vi "X682 Chassis Connectivity Tester Program Ver1.0.0.0.vi"() -> ()   [LabVIEW 2017]
uses:
  Ctrls/MainStep.ctl
  Ctrls/AllControls.ctl
  <vilib>/Utility/miscctls.llb/LVRowAndColumnTypeDef.ctl
  ComVIS/Files/Ini/WriteIniFiles_ByVarient.vi
  <instrlib>/GPP/GPP.lvlib
panel:
  in  "Recipe":string(combo)
  in  "MES Status":bool
  in  "maintenance":bool
  in  "mode":enum32{"Production mode", "Engineering mode"}(tab)
  out "Fail resume":bool caption="TotalResult"
  out "Table":string[][](table)
  out "LogInfo":string caption="Log"
  in  "AlarmData":i32(listbox)=-1
  out "Device state":bool caption="TotalResult"
  out "CT":dbl format="%#_3f"
  in  "ProductID:":string
  in  "TestInfo":T1 {"Yield" format="%#_g%"}
  out "MES_Status":string
  out "TestMode":string
  in  "Stop":bool
  in  "Start":bool
  in  "Exit":bool
  in  "Login":bool
  out "Login_status":string="Operator:Operator"
  out "OpenStatus":string
  in  "error in (no error)":errorcluster caption="错误输入（无错误）"
  # "Dyson X682 Chassis Connectivity Tester"
  # "Waiting Barcode scanning"
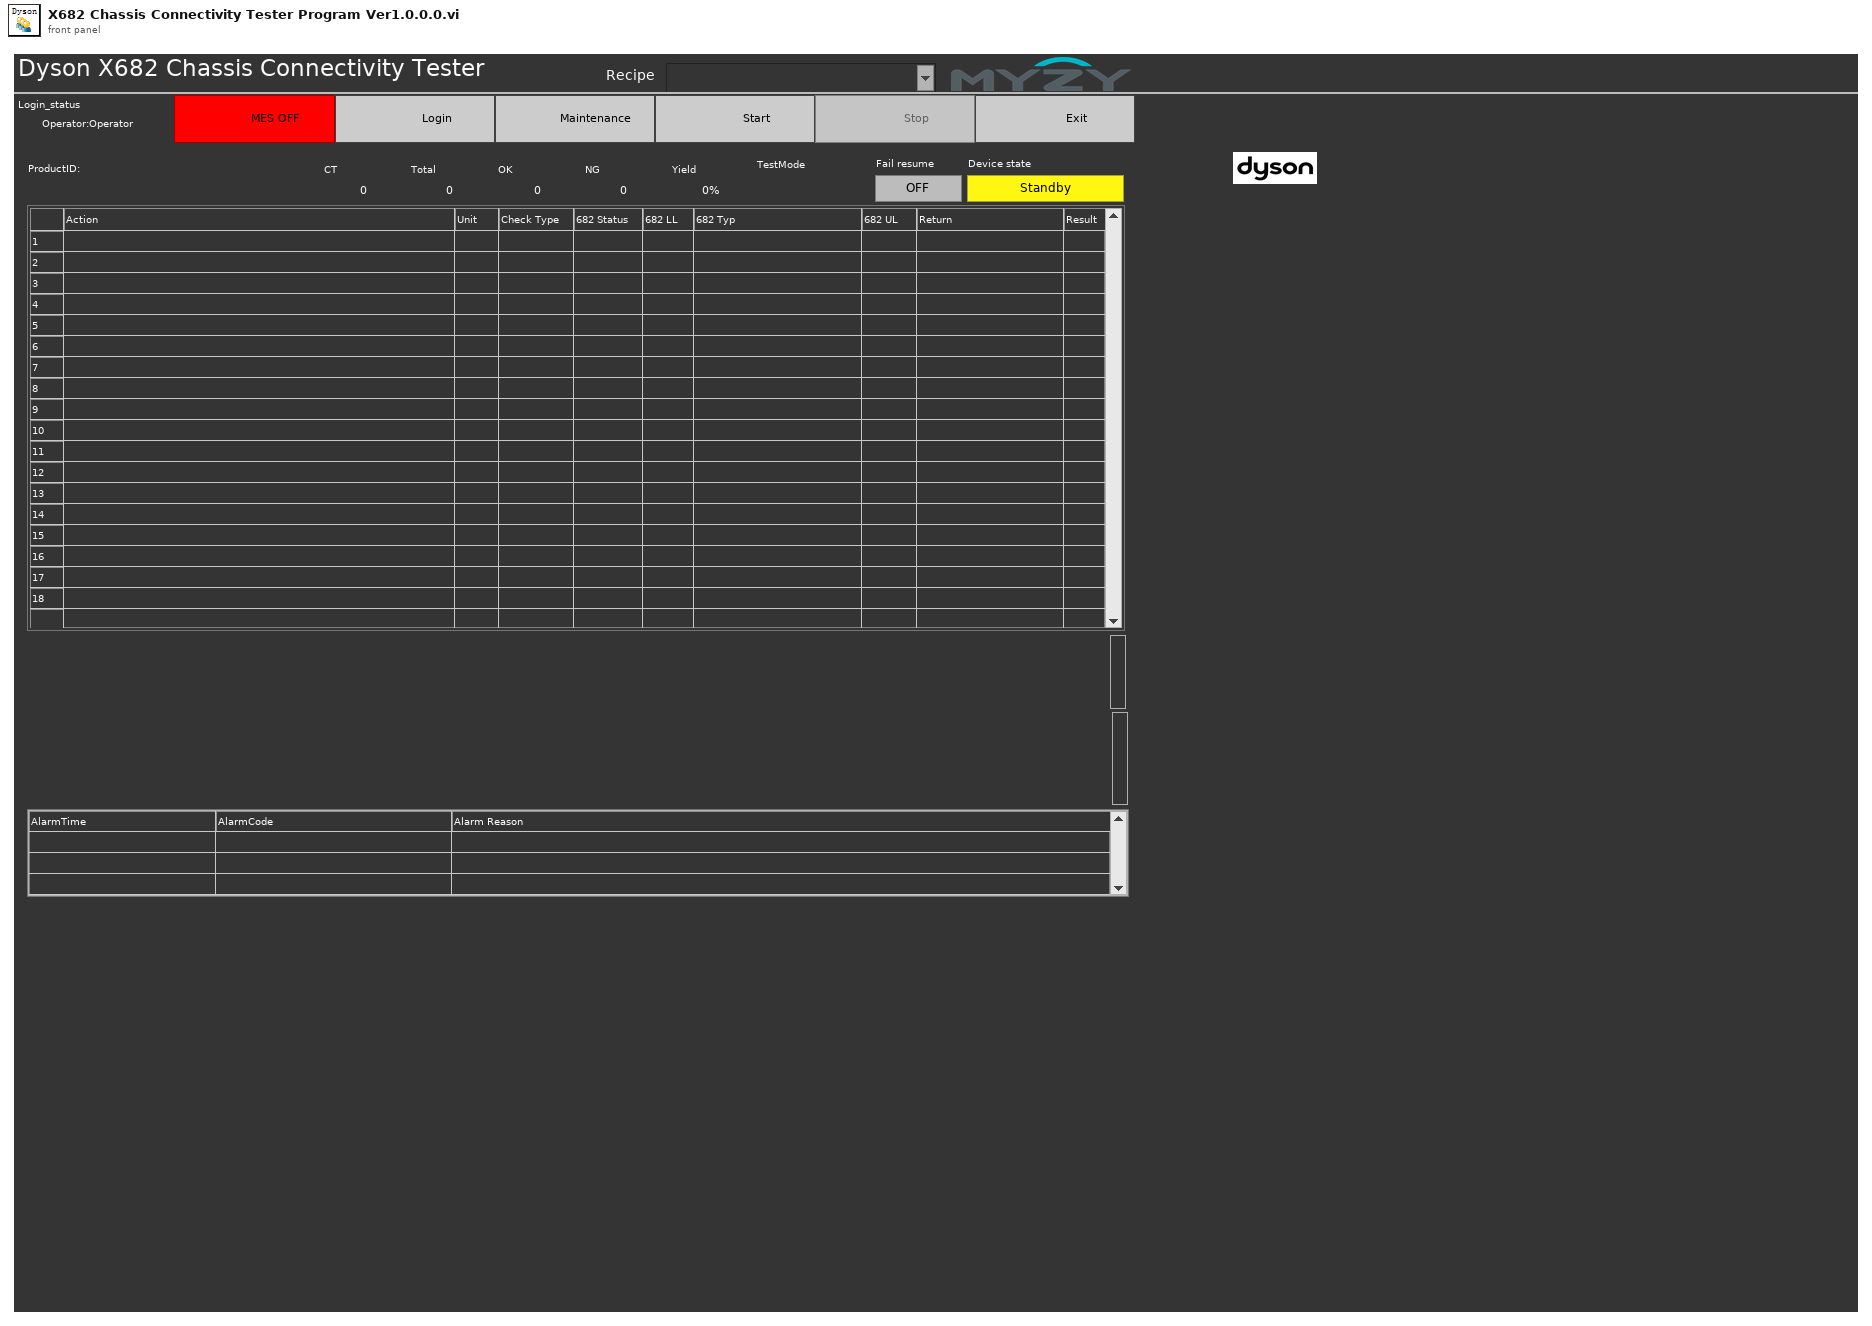
[diagram p1: front panel]
types:
  T1 = cluster{"Total":i32, "OK":i32, "NG":i32, "Yield":dbl}
  T2 = typedef "MainStep.ctl" = enum16{"Initialize", "ReadAllFiles", "ResetHardware", "Run", "Exit"}
  T3 = typedef "AllControls.ctl" = cluster{"MainVI":refnum<vi>, "AlarmInfo":refnum<vi>, "Log":refnum<vi>, "Current CT":refnum<vi>, "ProductID":refnum<vi>, "Device state":refnum<vi>, "MES":refnum<vi>, "mode":refnum<vi>, "TestInfo":refnum<vi>, "SubPnl":refnum<vi>, "Table":refnum<vi>, "MES bool":refnum<vi>, "TestMode":refnum<vi>, "Recipe":refnum<vi>, "Fail resume":refnum<vi>, "LogIn":refnum<vi>, "Start":refnum<vi>, "Maintenance":refnum<vi>, "Stop":refnum<vi>, "Exit":refnum<vi>}
  T4 = enum32{"Invalid", "Standard", "Closed", "Hidden", "Minimized", "Maximized"}
  T5 = enum16{"Ini", "Standby", "Running", "Engineering"}
  T6 = typedef "LVRowAndColumnTypeDef.ctl" = cluster{"Row":i32, "Column":i32}
  T7 = enum32{"invalid app kind", "Development System", "Run Time System", "Student Edition", "Embedded LabVIEW", "Evaluation", "Custom"}
  T8 = typedef "amc_Message Queue.ctl" = refnum<queue>
  T9 = typedef "HD Config.ctl" = cluster{" PC":cluster{"PC Address":u8[], "PC Port":i32}, "FCO":cluster{"COM":refnum<visa-resource-name>, "Baudrate":u32}, "DC Power ":cluster{"COM":refnum<visa-resource-name>, "Baudrate":u32}, "PW3336":cluster{"COM":refnum<visa-resource-name>, "Baudrate":u32}, "Lefoo":cluster{"COM":refnum<visa-resource-name>, "Baudrate":u32}, "Tempt&Hum":cluster{"COM":refnum<visa-resource-name>, "Baudrate":u32}, "DIPC":cluster{"COM":refnum<visa-resource-name>}, "Daemon":cluster{"IP Address":string, "Port":u16, "Retry":u16}, "URAT":cluster{"COM":refnum<visa-resource-name>, "Baudrate":u32}, "Fail_resume_mode":bool, "GRR":bool}
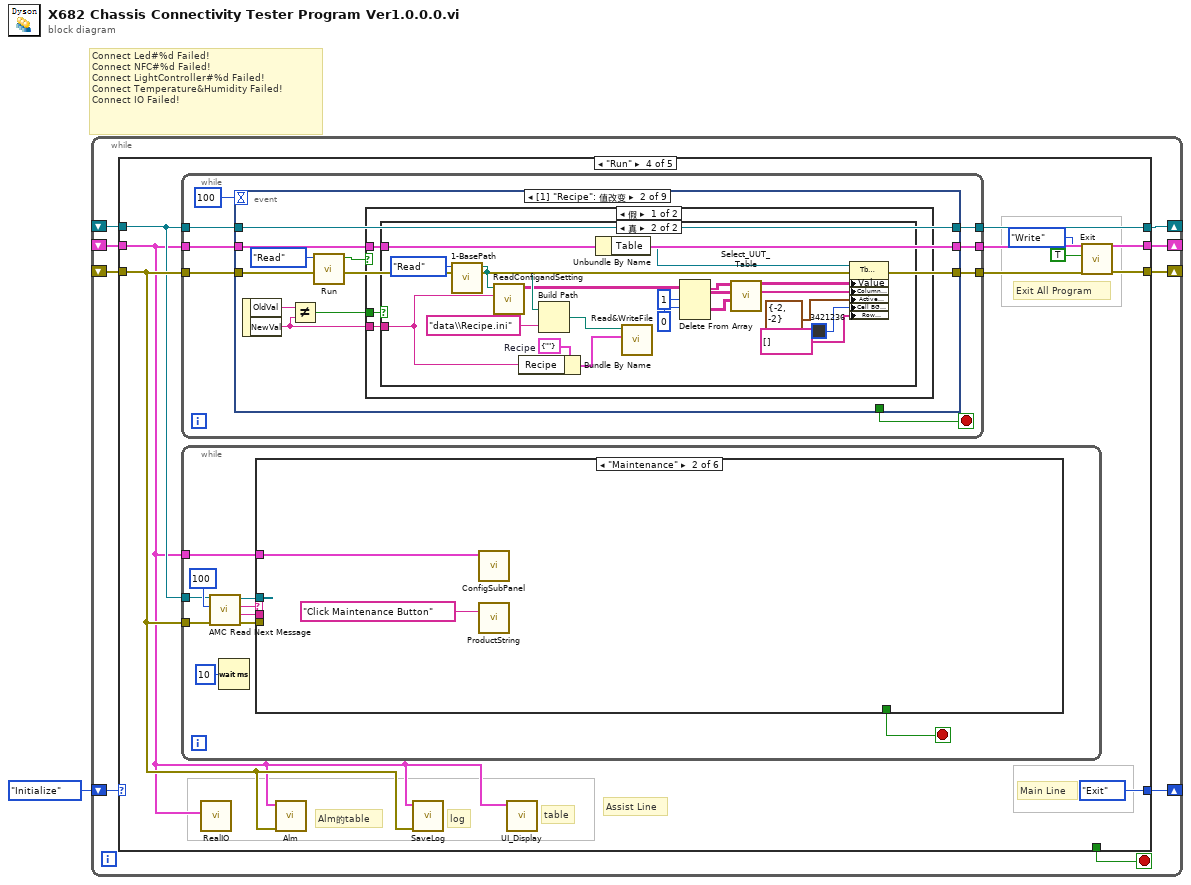
[diagram p0: block diagram]
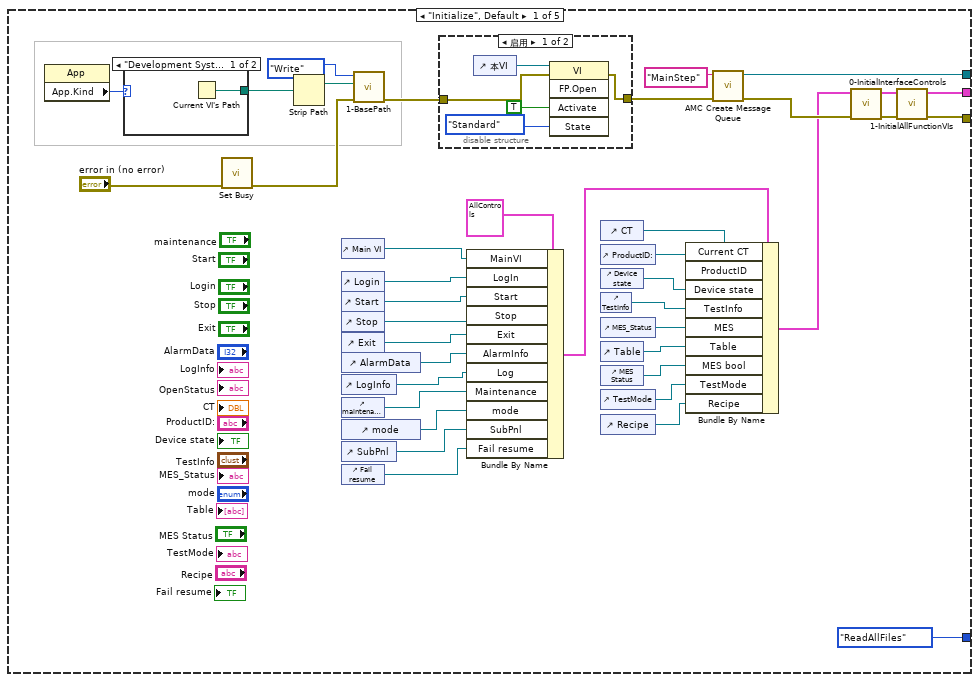
[diagram p2: hidden frame]
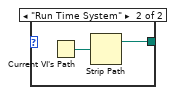
[diagram p4: hidden frame]
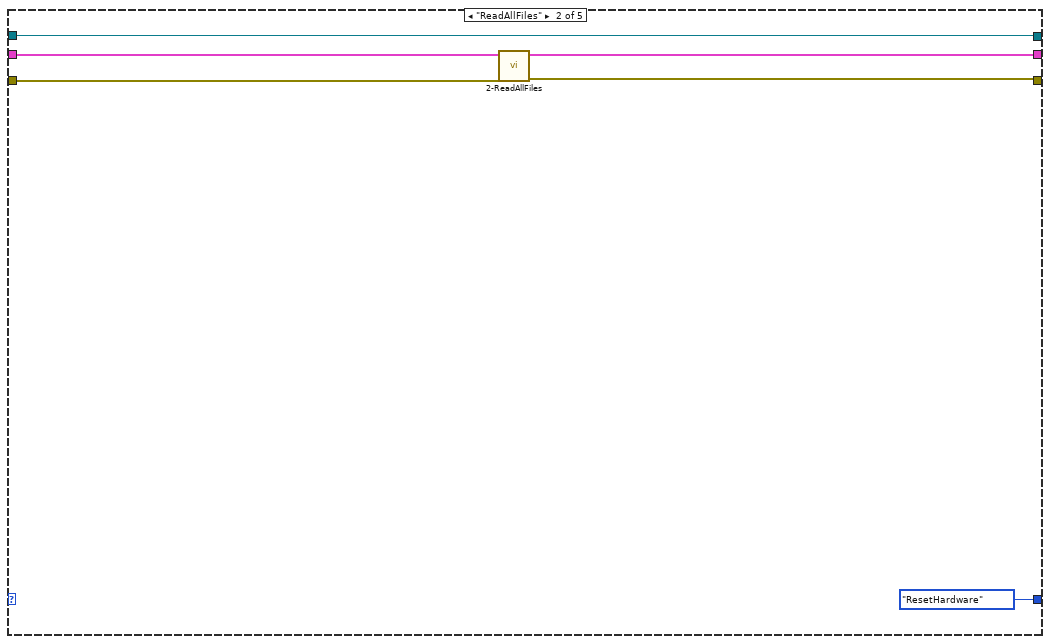
[diagram p5: hidden frame]
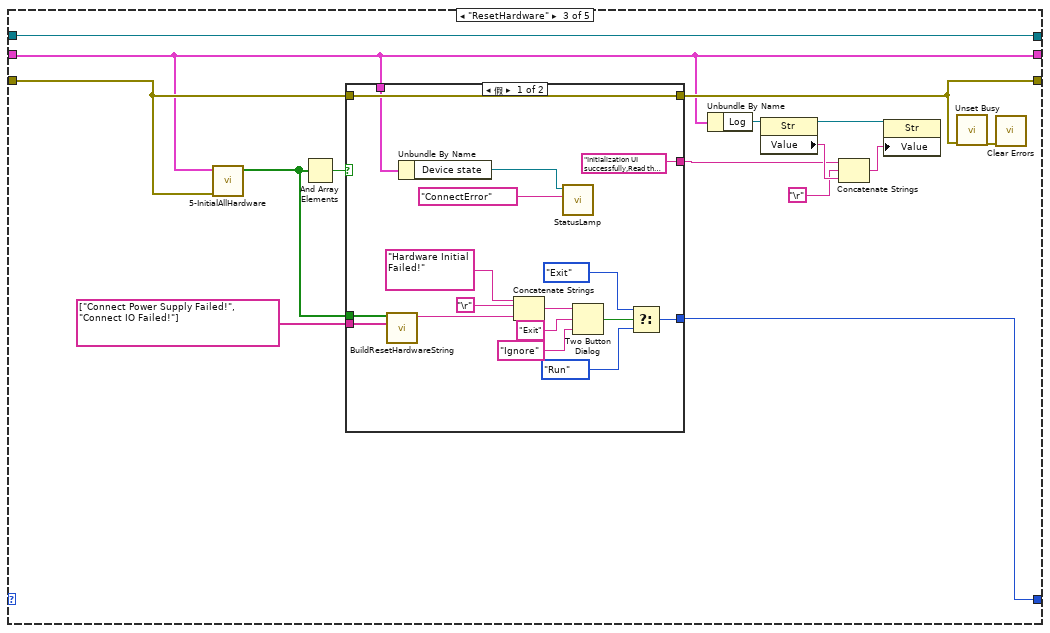
[diagram p6: hidden frame]
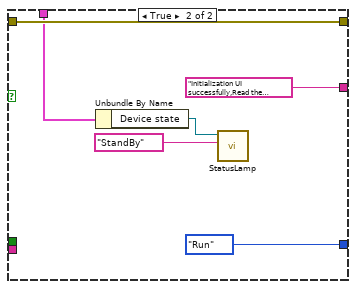
[diagram p7: hidden frame]
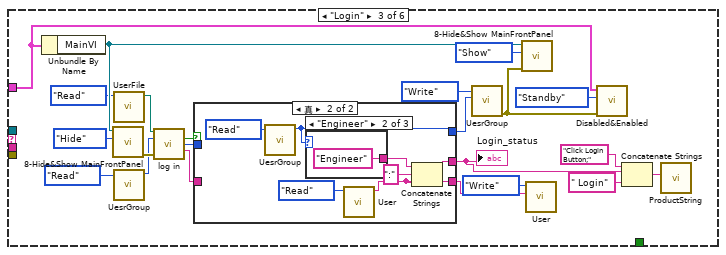
[diagram p9: hidden frame]
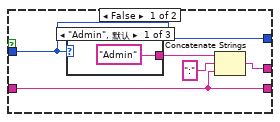
[diagram p10: hidden frame]
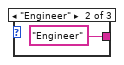
[diagram p11: hidden frame]
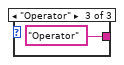
[diagram p12: hidden frame]
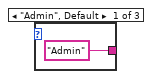
[diagram p13: hidden frame]
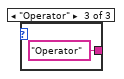
[diagram p14: hidden frame]
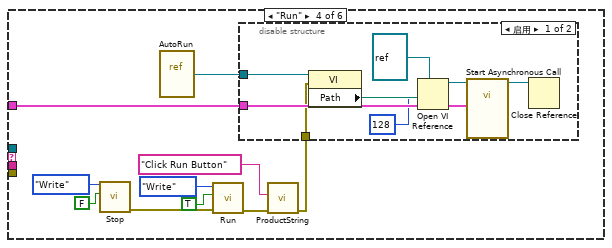
[diagram p15: hidden frame]
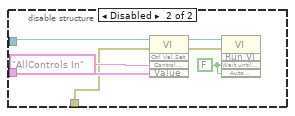
[diagram p16: hidden frame]
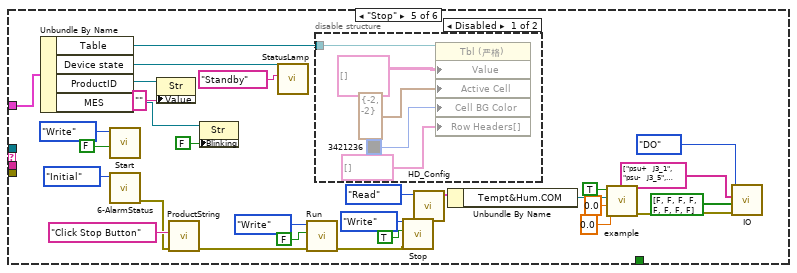
[diagram p17: hidden frame]
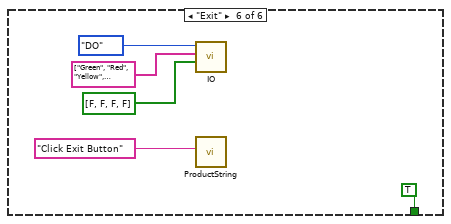
[diagram p19: hidden frame]
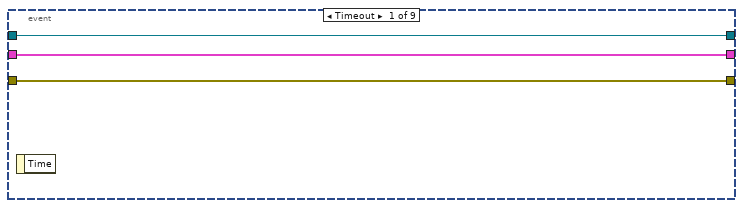
[diagram p20: hidden frame]
diagram:
  # "Connect Led#%d Failed!\nConnect NFC#%d Failed!\nConnect LightController#%d Failed!\nConnect Temperature&Humidity Failed!\nConnect IO Failed!"
  n1 = while {
    shift-right: [w9] -> _
    shift-left: MainStep."Initialize" -> [w10]
    shift-right: [w7] -> _
    shift-left: _ -> [w2]
    shift-right: [w5] -> _
    shift-left: _ -> [w3]
    shift-right: [w6] -> _
    shift-left: _ -> [w4]
    stop <- w8 stop-if-true
    n2 = case shown="\"Run\"" w10 {
      tunnel: [MainStep."ReadAllFiles" MainStep."ResetHardware" w79 MainStep."Exit" MainStep."Exit"] -> w9
      tunnel: [_ _ _ _ TRUE] -> w8
      tunnel: [w36 w59 w75 w106 w359] -> w7
      tunnel: [w44 w63 w78 w111 _] -> w6
      tunnel: [w37 w61 w73 w110 w357] -> w5
      tunnel: w4 -> [_ w63 w78 w104 w360]
      tunnel: w3 -> [_ w62 w73 w103 w357]
      tunnel: w2 -> [_ w60 w76 w105 w358]
      frame "Initialize", Default {
        n3 = property class="App"() -> ("App.Kind"=w48:T7)  [unwired: 2 in, 2 out]
        n4 = case shown="\"Development System\", 默认" w48 {
          tunnel: [w56 w57] -> w47
          frame "Development System", Default {
            n5 = Current VI's Path() -> (path=w56:path)
          }
          frame "Run Time System" {
            n6 = Current VI's Path() -> (path=w58:path)
            n7 = Strip Path(path=w58) -> (stripped path=w57:path)  [unwired: 1 out]
          }
        }
        n8 = call <vilib>:"Set Busy.vi"("error in (no error)"="error in (no error)") -> ("error out"=w16:errorcluster)  [unwired: 9 in, 1 out]
        n9 = Strip Path(path=w47) -> (stripped path=w17:path)  [unwired: 1 out]
        n10 = control-ref of="Main VI"() -> (w34:refnum<vi>)
        n11 = control-ref of="Login"() -> (w24:refnum<vi>)
        n12 = control-ref of="Start"() -> (w25:refnum<vi>)
        n13 = control-ref of="Stop"() -> (w26:refnum<vi>)
        n14 = control-ref of="Exit"() -> (w27:refnum<vi>)
        n15 = control-ref of="AlarmData"() -> (w42:refnum<vi>)
        n16 = control-ref of="LogInfo"() -> (w41:refnum<vi>)
        n17 = control-ref of="maintenance"() -> (w22:refnum<vi>)
        n18 = control-ref of="mode"() -> (w23:refnum<vi>)
        n19 = control-ref of="SubPnl"() -> (w21:refnum<vi>)
        n20 = control-ref of="Fail resume"() -> (w11:refnum<vi>)
        n21 = call "1-BasePath.vi"("error in (no error)"=w16, "Path In"=w17, "Step"=enum16{"Initial", "Write", "Read"}."Write") -> ("error out"=w15:errorcluster)  [unwired: 7 in, 1 out]
        n22 = disable-structure shown="启用" {
          disable-tunnel: w15 -> [w52 w55]
          disable-tunnel: [w50 w55] -> w45
          frame Enabled {
            n23 = control-ref of="本VI"() -> (w54:refnum<vi>)
            n24 = invoke class="VI" method="FP.Open"(reference=w54, error in=w52, "Activate"=TRUE ("激活？"), "State"=T4."Standard" ("状态")) -> (error out=w50:errorcluster)  [unwired: 1 in, 4 out]
          }
          frame Disabled {
          }
        }
        n25 = Bundle By Name(cluster=T3 {"MainVI"=refnum, "AlarmInfo"=refnum, "Log"=refnum, "Current CT"=refnum, "ProductID"=refnum, "Device state"=refnum, "MES"=refnum, "mode"=refnum, "TestInfo"=refnum, "SubPnl"=refnum, "Table"=refnum, "MES bool"=refnum, "TestMode"=refnum, "Recipe"=refnum, "Fail resume"=refnum, "LogIn"=refnum, "Start"=refnum, "Maintenance"=refnum, "Stop"=refnum, "Exit"=refnum}, "MainVI"=w34, "LogIn"=w24, "Start"=w25, "Stop"=w26, "Exit"=w27, "AlarmInfo"=w42, "Log"=w41, "Maintenance"=w22, "mode"=w23, "SubPnl"=w21, "Fail resume"=w11) -> (w33:T3)
        n26 = control-ref of="CT"() -> (w30:refnum<vi>)
        n27 = control-ref of="ProductID:"() -> (w31:refnum<vi>)
        n28 = control-ref of="Device state"() -> (w32:refnum<vi>)
        n29 = control-ref of="TestInfo"() -> (w29:refnum<vi>)
        n30 = control-ref of="MES_Status"() -> (w28:refnum<vi>)
        n31 = control-ref of="Table"() -> (w19:refnum<vi>)
        n32 = control-ref of="MES Status"() -> (w14:refnum<vi>)
        n33 = control-ref of="TestMode"() -> (w13:refnum<vi>)
        n34 = control-ref of="Recipe"() -> (w12:refnum<vi>)
        n35 = Bundle By Name(cluster=w33, "Current CT"=w30, "ProductID"=w31, "Device state"=w32, "TestInfo"=w29, "MES"=w28, "Table"=w19, "MES bool"=w14, "TestMode"=w13, "Recipe"=w12) -> (w20:T3)
        n36 = call "AMC Create Message Queue.vi"("error in (no error)"=w45, "Message Queue Name"="MainStep" ("Message queue name (unnamed)")) -> ("error out"=w40:errorcluster, "Message Queue out"=w44:T8)  [unwired: 3 in, 5 out]
        n37 = call "0-InitialInterfaceControls.vi"("error in (no error)"=w40, "AllControls IN"=w20) -> ("error out"=w39:errorcluster, "AllControls Out"=w38:T3)  [unwired: 8 in]
        n38 = call "1-InitialAllFunctionVIs.vi"("error in (no error)"=w39, "AllControls IN"=w38) -> ("error out"=w36:errorcluster, "AllControls Out"=w37:T3)  [unwired: 8 in]
      }
      frame "ReadAllFiles" {
        n39 = call "2-ReadAllFiles.vi"("error in (no error)"=w60, "AllControls IN"=w62) -> ("error out"=w59:errorcluster, "AllControls Out"=w61:T3)  [unwired: 8 in]
      }
      frame "ResetHardware" {
        n40 = call "5-InitialAllHardware.vi"("error in (no error)"=w76, "AllControls IN"=w73) -> ("InitalResult"=w77:bool[])  [unwired: 9 in]
        n41 = And Array Elements(Boolean array=w77) -> (logical AND=w65:bool)
        n42 = case shown="假" w65 {
          tunnel: [w87 MainStep."Run"] -> w79
          tunnel: w76 -> [w96 w101]
          tunnel: string[] ["Connect Power Supply Failed!", "Connect IO Failed!"] -> [w85 _]
          tunnel: w77 -> [w86 _]
          tunnel: [w96 w101] -> w75
          tunnel: ["Initialization UI successfully,Read the configuration parameter successfully,Initialize hardware failure" ("值") "Initialization UI successfully,Read the configuration parameter successfully,Initialize hardware successfully" ("值")] -> w69
          tunnel: w73 -> [w80 w99]
          frame False {
            n43 = call "BuildResetHardwareString.vi"("String"=w85, "Error"=w86) -> ("DataOut"=w84:string)  [unwired: 9 in]
            n44 = Unbundle By Name(w80) -> ("Device state"=w81:refnum<vi>)
            n45 = Concatenate Strings("Hardware Initial Failed!" ("caption"), "\r", w84) -> (w94:string)
            n46 = call "StatusLamp.vi"("State"="ConnectError", "Boolean输入"=w81) -> ()  [unwired: 9 in, 1 out]
            n47 = Two Button Dialog(message=w94, 1:"Ignore" ("F按钮名称（“取消”）"), 2:"Exit" ("T按钮名称（“确定”）")) -> (T button?=w90:bool)
            n48 = Select(t=MainStep."Exit", s=w90, f=MainStep."Run") -> (s? t:f=w87:T2)
          }
          frame True {
            n49 = Unbundle By Name(w99) -> ("Device state"=w97:refnum<vi>)
            n50 = call "StatusLamp.vi"("State"="StandBy", "Boolean输入"=w97) -> ()  [unwired: 9 in, 1 out]
          }
        }
        n51 = Unbundle By Name(w73) -> ("Log"=w70:refnum<vi>)
        n52 = property class="Str"(reference=w70) -> (reference out=w68:refnum<vi>, "Value"=w72:string)  [unwired: 1 in, 1 out]
        n53 = Concatenate Strings(w69, "\r", w72) -> (w67:string)
        n54 = property class="Str"(reference=w68, "Value"=w67) -> ()  [unwired: 1 in, 2 out]
        n55 = call <vilib>:"Unset Busy.vi"("error in (no error)"=w75) -> ("error out"=w74:errorcluster)  [unwired: 10 in]
        n56 = call <vilib>:"Clear Errors.vi"("error in (no error)"=w74) -> ()  [unwired: 5 in, 2 out]
      }
      frame "Run" {
        # "Alm的table"
        # "log"
        # "table"
        # "Exit All Program"
        # "Assist Line"
        # "Main Line"
        n57 = while {
          tunnel: w104 -> [w236]
          tunnel: w103 -> [w235]
          tunnel: w105 -> [w234]
          tunnel: [w233] -> w111
          tunnel: [w232] -> w110
          tunnel: [w231] -> w107
          stop <- w230 stop-if-true
          n58 = event shown="[1] \"Recipe\": 值改变" {
            selector: _ -> [_ _ _ _ _ _ _ _ _]
            dyn-events: _ -> [_ _ _ _ _ _ _ _ _]
            timeout: 100 -> [_ _ _ _ _ _ _ _ _]
            tunnel: w236 -> [w239 w247 w272 w278 w290 w315 w329 w338 w345]
            tunnel: w235 -> [w238 w242 w270 w277 w288 w313 w327 w340 w350]
            tunnel: w234 -> [w237 w246 w271 w280 w289 w314 w328 w337 w346]
            tunnel: [w239 w247 w272 w278 w290 w315 w329 w338 w345] -> w233
            tunnel: [w238 w242 w270 w277 w288 w313 w327 w340 w350] -> w232
            tunnel: [w237 w246 w271 w280 w289 w314 w328 w337 w346] -> w231
            tunnel: [_ _ _ _ _ _ _ w336 w349] -> w230
            event Timeout {
              n59 = event-data() -> ()  [unwired: 1 in, 1 out]
            }
            event "Recipe": Value Change {
              n60 = event-data() -> ("OldVal"=w245:string, "NewVal"=w243:string)  [unwired: 1 in]
              n61 = Not Equal?(x=w245, y=w243) -> (x != y?=w244:bool)
              n62 = call "Run.vi"("Step"=enum16{"Initial", "Write", "Read"}."Read") -> ("Run Out"=w240:bool)  [unwired: 9 in, 1 out]
              n63 = case shown="假" w240 {
                tunnel: w244 -> [w250 _]
                tunnel: w243 -> [w249 _]
                tunnel: w242 -> [w248 _]
                frame False {
                  n64 = case shown="真" w250 {
                    tunnel: w249 -> [_ w264]
                    tunnel: w248 -> [_ w252]
                    frame False {
                    }
                    frame True {
                      w265 = cluster{"Recipe":string} {"Recipe"=""}  # Recipe
                      n65 = call "1-BasePath.vi"("Step"=enum16{"Initial", "Write", "Read"}."Read") -> ("Path Out"=w266:path)  [unwired: 9 in, 1 out]
                      n66 = call "ReadConfigandSetting.vi"("Recipe"=w264, "Path Out"=w266) -> ("TableData"=w253:string[][])  [unwired: 7 in, 2 out]
                      n67 = Bundle By Name(cluster=w265, "Recipe"=w264) -> (w263:cluster{"Recipe":string})
                      n68 = Build Path(base path=w266, name or relative path="data\\Recipe.ini") -> (appended path=w268:path)
                      n69 = Unbundle By Name(w252) -> ("Table"=w251:refnum<vi>)
                      n70 = call-poly "Read&WriteFile.vi"("Variant"=w263, "path"=w268) -> ()  [unwired: 9 in, 1 out]
                      n71 = Delete From Array(array=w253, length=1 ("长度"), index (row)=0 ("索引 (行)")) -> (deleted portion=w261:string[][], array with subset deleted=w259:string[][])  [unwired: 1 in]
                      n72 = call "Select_UUT_Table.vi"("all Title"=w261, "all Table"=w259) -> ("Title"=w260:string[], "Table"=w262:string[][])  [unwired: 8 in]
                      n73 = property class="Tbl (严格)"(reference=w251, "Value"=w262, "Column Headers[]"=w260, "Active Cell"=T6 {"Row"=-2, "Column"=-2} ("活动单元格:活动单元格"), "Cell BG Color"=u32 3421236, "Row Headers[]"=string[] [] ("Row Header Strings[]")) -> ()  [unwired: 1 in, 2 out]
                    }
                  }
                }
                frame True {
                }
              }
            }
            event "Login": Value Change {
              n74 = event-data() -> ("NewVal"=w273:bool)  [unwired: 1 in]
              n75 = case shown="真" w273 {
                tunnel: w272 -> [w276 _]
                tunnel: w271 -> [w275 _]
                frame True {
                  n76 = call "AMC Send Local Message.vi"("error in (no error)"=w275, "Message Name"="Login", "Message Queue in"=w276) -> ()  [unwired: 7 in, 2 out]
                }
                frame False {
                }
              }
            }
            event "maintenance": Value Change {
              n77 = event-data() -> ("NewVal"=w281:bool)  [unwired: 1 in]
              n78 = Unbundle By Name(w277) -> ("mode"=w279:refnum<vi>)
              n79 = case shown="真" w281 {
                tunnel: w279 -> [w287 _]
                tunnel: w278 -> [w284 _]
                tunnel: w277 -> [w283 _]
                frame True {
                  n80 = call "AMC Send Local Message.vi"("Message Name"="Maintenance", "Message Queue in"=w284) -> ()  [unwired: 8 in, 2 out]
                  n81 = property class="TabCtl (严格)"(reference=w287, "Value"=enum32{"Production mode", "Engineering mode"}."Engineering mode" ("值")) -> ()  [unwired: 1 in, 2 out]
                  n82 = call "Disabled&Enabled.vi"("Mode in"=T5."Engineering", "AllControls In"=w283) -> ()  [unwired: 9 in, 1 out]
                }
                frame False {
                }
              }
            }
            event "Start": Value Change {
              n83 = event-data() -> ("NewVal"=w291:bool)  [unwired: 1 in]
              n84 = case shown="真" w291 {
                tunnel: w290 -> [w296 _]
                tunnel: w289 -> [w295 _]
                tunnel: w288 -> [w292 _]
                frame True {
                  n85 = call "AMC Send Local Message.vi"("error in (no error)"=w295, "Message Name"="Run", "Message Queue in"=w296) -> ()  [unwired: 7 in, 2 out]
                  n86 = call "Disabled&Enabled.vi"("Mode in"=T5."Running", "AllControls In"=w292) -> ()  [unwired: 9 in, 1 out]
                }
                frame False {
                }
              }
            }
            event "MES Status": Value Change {
              n87 = event-data() -> ("NewVal"=w297:bool)  [unwired: 1 in]
              n88 = Unbundle By Name(w313) -> ("MES bool"=w306:refnum<vi>, "TestMode"=w298:refnum<vi>)
              n89 = call "HD_Config.vi"("Step"=enum16{"Initial", "Write", "Read"}."Read") -> ("HD Config out"=w305:T9)  [unwired: 9 in, 1 out]
              n90 = Unbundle By Name(w305) -> ("Fail_resume_mode"=w302:bool, "GRR"=w300:bool)
              n91 = Not(x=w297) -> (.not. x?=w304:bool)
              n92 = Or(x=w302, y=w304) -> (x .or. y?=w303:bool)
              n93 = case shown="真" w300 {
                tunnel: w303 -> [w317 _]
                tunnel: [w316 "GRR"] -> w301
                frame False {
                  n94 = case shown="假" w317 {
                    tunnel: ["Production" "Engineering"] -> w316
                    frame False {
                    }
                    frame True {
                    }
                  }
                }
                frame True {
                }
              }
              n95 = property class="Str"(reference=w298, "Value"=w301) -> ()  [unwired: 1 in, 2 out]
              n96 = Select(t="MES ON", s=w297, f="MES OFF") -> (s? t:f=w307:string)
              n97 = case shown="\"MES ON\", 默认" w307 {
                selector: w307 -> [w321 w324]
                tunnel: [TRUE FALSE] -> w309
                tunnel: [w321 w324] -> w310
                tunnel: [cluster{u32, u32}[] [{6618880, 6618880}] cluster{u32, u32}[] [{16711680, 16711680}]] -> w308
                frame "MES ON", Default {
                }
                frame "MES OFF" {
                }
              }
              n98 = property on="属性节点" class="Bool (严格)"(reference=w306, "Value"=w309, "Colors [4]"=w308, "BoolText.Text"=w310) -> ()  [unwired: 1 in, 2 out]
            }
            event "Stop": Value Change {
              n99 = event-data() -> ("NewVal"=w330:bool)  [unwired: 1 in]
              n100 = case shown="真" w330 {
                tunnel: w329 -> [w335 _]
                tunnel: w328 -> [w334 _]
                tunnel: w327 -> [w331 _]
                frame True {
                  n101 = call "AMC Send Local Message.vi"("error in (no error)"=w334, "Message Name"="Stop", "Message Queue in"=w335) -> ()  [unwired: 7 in, 2 out]
                  n102 = call "Disabled&Enabled.vi"("Mode in"=T5."Standby", "AllControls In"=w331) -> ()  [unwired: 9 in, 1 out]
                }
                frame False {
                }
              }
            }
            event "Exit": Value Change {
              n103 = event-data() -> ("NewVal"=w339:bool)  [unwired: 1 in]
              n104 = case shown="真" w339 {
                tunnel: w338 -> [_ w344]
                tunnel: w337 -> [_ w343]
                tunnel: [_ TRUE] -> w336
                frame False {
                }
                frame True {
                  n105 = call "AMC Send Local Message.vi"("error in (no error)"=w343, "Message Name"="Exit", "Message Queue in"=w344) -> ()  [unwired: 7 in, 2 out]
                }
              }
            }
            event Panel Close? {
              n106 = event-data() -> ()  [unwired: 1 in, 1 out]
              n107 = Two Button Dialog(message="Are you sure to Exit system?") -> (T button?=w348:bool)  [unwired: 2 in]
              n108 = case shown="假" w348 {
                selector: w348 -> [w352 w353]
                tunnel: [w352 w353] -> w349
                frame False {
                }
                frame True {
                }
              }
              n109 = Not(x=w349) -> (.not. x?=w351:bool)
              n110 = event-data("Discard?"=w351) -> ()  [unwired: 1 in, 1 out]
            }
          }
        }
        n111 = while {
          tunnel: w103 -> [w122]
          tunnel: w105 -> [w119]
          tunnel: w104 -> [w116]
          stop <- w113 stop-if-true
          n112 = call "AMC Read Next Message.vi"("error in (no error)"=w119, "timeout (1ms)"=100 ("Timeout"), "Message Queue in"=w116) -> ("error out"=w118:errorcluster, "Message Value"=w114:string, "Message Name"=w117:string, "Message Queue out"=w115:T8)  [unwired: 1 in, 4 out]
          n113 = Wait (ms)(milliseconds to wait=u32 10 ("毫秒倍数")) -> ()  [unwired: 1 out]
          n114 = case shown="\"Maintenance\"" w117 {
            tunnel: w122 -> [_ w124 w132 w167 w217 _]
            tunnel: w118 -> [_ _ _ _ _ _]
            tunnel: [_ _ _ _ _ TRUE] -> w113
            tunnel: w115 -> [_ _ _ _ _ _]
            tunnel: w114 -> [_ _ _ _ _ _]
            frame "Null", Default {
            }
            frame "Maintenance" {
              n115 = call "ConfigSubPanel.vi"("AllControls"=w124) -> ()  [unwired: 11 in]
              n116 = call "ProductString.vi"("String"="Click Maintenance Button" ("值")) -> ()  [unwired: 10 in, 1 out]
            }
            frame "Login" {
              n117 = Unbundle By Name(w132) -> ("MainVI"=w145:refnum<vi>)
              n118 = call "8-Hide&Show MainFrontPanel.vi"("Hide&Show"=enum16{"Hide", "Show"}."Hide", "This VI"=w145) -> ("error out"=w143:errorcluster)  [unwired: 9 in]
              n119 = call "UserFile.vi"("Step"=enum16{"Initial", "Write", "Read"}."Read") -> ("UserPath out"=w142:path)  [unwired: 9 in, 1 out]
              n120 = call "UesrGroup.vi"("Step"=enum16{"Initial", "Write", "Read"}."Read") -> ("User group out"=w125:enum16{"Operator", "Engineer", "Admin"})  [unwired: 9 in, 1 out]
              n121 = call "log in.vi"("路径"=w142, "UserGroups in"=w125, "error in (no error)"=w143) -> ("Giveup?"=w140:bool, "UserGroups"=w139:enum16{"Operator", "Engineer", "Admin"}, "User"=w138:string)  [unwired: 8 in, 2 out]
              n122 = case shown="真" w140 {
                tunnel: [w148 w155] -> w134
                tunnel: [w149 w159] -> w128
                tunnel: [w147 w157] -> w136
                tunnel: w139 -> [w147 _]
                tunnel: w138 -> [w148 _]
                frame False {
                  n123 = case shown="\"Admin\", 默认" w147 {
                    tunnel: ["Admin" "Engineer" "Operator"] -> w151
                    frame "Admin", Default {
                    }
                    frame "Engineer" {
                    }
                    frame "Operator" {
                    }
                  }
                  n124 = Concatenate Strings(w151, ":" ("字符串"), w148) -> (w149:string)
                }
                frame True {
                  n125 = call "UesrGroup.vi"("Step"=enum16{"Initial", "Write", "Read"}."Read") -> ("User group out"=w157:enum16{"Operator", "Engineer", "Admin"})  [unwired: 9 in, 1 out]
                  n126 = case shown="\"Engineer\"" w157 {
                    tunnel: ["Admin" "Engineer" "Operator"] -> w161
                    frame "Admin", Default {
                    }
                    frame "Engineer" {
                    }
                    frame "Operator" {
                    }
                  }
                  n127 = call "User.vi"("Step"=enum16{"Initial", "Write", "Read"}."Read") -> ("User out"=w155:string)  [unwired: 9 in, 1 out]
                  n128 = Concatenate Strings(w161, ":" ("字符串"), w155) -> (w159:string)
                }
              }
              "Login_status" <- w128
              n129 = call "UesrGroup.vi"("User group in"=w136, "Step"=enum16{"Initial", "Write", "Read"}."Write") -> ("错误输出"=w131:errorcluster)  [unwired: 8 in, 1 out]
              n130 = call "8-Hide&Show MainFrontPanel.vi"("error in (no error)"=w131, "Hide&Show"=enum16{"Hide", "Show"}."Show", "This VI"=w145) -> ()  [unwired: 8 in, 1 out]
              n131 = call "User.vi"("User in"=w134, "Step"=enum16{"Initial", "Write", "Read"}."Write") -> ()  [unwired: 8 in, 2 out]
              n132 = call "Disabled&Enabled.vi"("error in (no error)"=w131, "Mode in"=T5."Standby", "AllControls In"=w132) -> ()  [unwired: 8 in, 1 out]
              n133 = Concatenate Strings("Click Login Button;" ("String"), w128, " Login" ("字符串")) -> (w129:string)
              n134 = call "ProductString.vi"("String"=w129) -> ()  [unwired: 10 in, 1 out]
            }
            frame "Run" {
              n135 = call "Stop.vi"("Stop In"=FALSE ("AutoStopping In"), "Step"=enum16{"Initial", "Write", "Read"}."Write") -> ("error out"=w173:errorcluster)  [unwired: 8 in, 1 out]
              n136 = vi-ref "AutoRun.vi"() -> (w165:refnum<vi>)
              n137 = call "Run.vi"("error in (no error)"=w173, "Run In"=TRUE ("AutoRun In"), "Step"=enum16{"Initial", "Write", "Read"}."Write") -> ("error out"=w168:errorcluster)  [unwired: 7 in, 1 out]
              n138 = call "ProductString.vi"("error"=w168, "String"="Click Run Button" ("值")) -> ("error  out"=w166:errorcluster)  [unwired: 9 in]
              n139 = disable-structure shown="启用" {
                disable-tunnel: w167 -> [w179 w185]
                disable-tunnel: w166 -> [w177 w183]
                disable-tunnel: w165 -> [w176 w184]
                frame Enabled {
                  n140 = property class="VI"(reference=w176, error in=w177) -> ("Path"=w182:path)  [unwired: 2 out]
                  n141 = Open VI Reference(type specifier VI Refnum (for type only)=refnum<vi> refnum ("application reference (local)"), vi path=w182, options=128) -> (vi reference=w180:refnum<vi>)  [unwired: 3 in, 1 out]
                  n142 = call-by-ref "Start Asynchronous Call"(reference=w180, "AllControls In"=w179) -> (reference out=w178:refnum<vi>)  [unwired: 12 in, 1 out]
                  n143 = Close Reference(reference=w178) -> ()  [unwired: 1 in, 1 out]
                }
                frame Disabled {
                  w186 = FALSE ("Wait Until Done")
                  n144 = invoke class="VI" method="Ctrl Val.Set"(reference=w184, error in=w183, "Control Name"="AllControls In", "Value"=w185) -> (reference out=w188:refnum<vi>, error out=w189:errorcluster)  [unwired: 1 in, 3 out]
                  n145 = invoke class="VI" method="Run VI"(reference=w188, error in=w189, "Wait until done"=w186, "Auto Dispose Ref"=w186) -> ()  [unwired: 1 in, 5 out]
                }
              }
            }
            frame "Stop" {
              n146 = Unbundle By Name(w217) -> ("Table"=w206:refnum<vi>, "Device state"=w214:refnum<vi>, "ProductID"=w216:refnum<vi>, "MES"=w201:refnum<vi>)
              n147 = call "Start.vi"("Start In"=FALSE, "Step"=enum16{"Initial", "Write", "Read"}."Write") -> ()  [unwired: 8 in, 2 out]
              n148 = call "6-AlarmStatus.vi"("Step"=enum16{"Initial", "Write", "Read"}."Initial") -> ("error out"=w202:errorcluster)  [unwired: 9 in, 1 out]
              n149 = property class="Str"(reference=w216, "Value"="") -> ()  [unwired: 1 in, 2 out]
              n150 = call "ProductString.vi"("error"=w202, "String"="Click Stop Button" ("值")) -> ("error  out"=w207:errorcluster)  [unwired: 9 in]
              n151 = property class="Str"(reference=w201, "Blinking"=FALSE ("闪烁")) -> ()  [unwired: 1 in, 2 out]
              n152 = call "StatusLamp.vi"("State"="Standby", "Boolean输入"=w214) -> ()  [unwired: 9 in, 1 out]
              n153 = call "Run.vi"("error in (no error)"=w207, "Run In"=FALSE ("AutoRun In"), "Step"=enum16{"Initial", "Write", "Read"}."Write") -> ("error out"=w212:errorcluster)  [unwired: 7 in, 1 out]
              n154 = disable-structure shown="Disabled" {
                disable-tunnel: w206 -> [w220 _]
                frame Disabled {
                  n155 = property class="Tbl (严格)"(reference=w220, "Value"=string[][] [] ("值"), "Active Cell"=T6 {"Row"=-2, "Column"=-2} ("活动单元格:活动单元格"), "Cell BG Color"=u32 3421236, "Row Headers[]"=string[] [] ("Row Header Strings[]")) -> ()  [unwired: 1 in, 2 out]
                }
                frame Enabled {
                }
              }
              n156 = call "Stop.vi"("error in (no error)"=w212, "Stop In"=TRUE ("AutoStopping In"), "Step"=enum16{"Initial", "Write", "Read"}."Write") -> ()  [unwired: 7 in, 2 out]
              n157 = call "HD_Config.vi"("Step"=enum16{"Initial", "Write", "Read"}."Read") -> ("HD Config out"=w197:T9)  [unwired: 9 in, 1 out]
              n158 = Unbundle By Name(w197) -> ("Tempt&Hum.COM"=w198:refnum<visa-resource-name>)
              n159 = call <instrlib>:"example.vi"("Current Level (A)"=0.0, "Voltage Level (V)"=0.0, "VISA resource name"=w198, "FLAG"=TRUE) -> ("error out"=w199:errorcluster)  [unwired: 4 in, 3 out]
              n160 = call "IO.vi"("错误常量"=w199, "DO DATA"=bool[] [FALSE, FALSE, FALSE, FALSE, FALSE, FALSE, FALSE, FALSE], "IO Name"=string[] ["psu+   J3_1", "psu-   J3_5", "UART1_3V3  J63_1", "UART1_TX   J63_5", "UART1_RX   J63_6", "UART1_GND  J63_10", "PSU S+ J3_1", "PSU S- J3_5"], "IO?"=enum16{"DI", "DO"}."DO") -> ()  [unwired: 6 in, 2 out]
            }
            frame "Exit" {
              n161 = call "IO.vi"("DO DATA"=bool[] [FALSE, FALSE, FALSE, FALSE], "IO Name"=string[] ["Green", "Red", "Yellow", "Buzzer"], "IO?"=enum16{"DI", "DO"}."DO") -> ()  [unwired: 7 in, 2 out]
              n162 = call "ProductString.vi"("String"="Click Exit Button" ("值")) -> ()  [unwired: 10 in, 1 out]
            }
          }
        }
        n163 = call "RealIO.vi"("AllControls Out"=w103) -> ()  [unwired: 11 in]
        n164 = call "Alm.vi"("error in (no error)"=w105, "AllControls Out"=w103) -> ()  [unwired: 10 in]
        n165 = call "SaveLog.vi"("错误输入（无错误）"=w105, "AllControls In"=w103) -> ()  [unwired: 9 in, 1 out]
        n166 = call "UI_Display.vi"("AllControls In"=w103) -> ()  [unwired: 11 in]
        n167 = call "Exit.vi"("error in (no error)"=w107, "Exit In"=TRUE, "Step"=enum16{"Initial", "Write", "Read"}."Write" ("step")) -> ("error out"=w106:errorcluster)  [unwired: 7 in, 1 out]
      }
      frame "Exit" {
        n168 = flat-sequence {
          tunnel: w358 -> [w363]
          tunnel: w357 -> [w369]
          frame #0 {
            n169 = call "ExitAllResource.vi"("error in (no error)"=w363) -> ("error out"=w364:errorcluster)  [unwired: 10 in]
            n170 = property class="App"(error in=w364) -> ("App.Kind"=w365:T7)  [unwired: 1 in, 2 out]
            n171 = case shown="\"Run Time System\"" w365 {
              frame "Development System", Default {
              }
              frame "Run Time System" {
                n172 = control-ref of="本VI"() -> (w366:refnum<vi>)
                n173 = invoke class="VI" method="FP.Close"(reference=w366) -> (error out=w367:errorcluster)  [unwired: 2 in, 2 out]
                n174 = call <vilib>:"Clear Errors.vi"("error in (no error)"=w367) -> ()  [unwired: 5 in, 2 out]
              }
            }
          }
          frame #1 {
            n175 = disable-structure shown="禁用" {
              frame Disabled {
                n176 = Quit LabVIEW(quit? (T)=TRUE) -> ()
              }
              frame Enabled {
              }
            }
            n177 = Unbundle By Name(w369) -> ("MainVI"=w368:refnum<vi>)
            n178 = Close Reference(reference=w368) -> ()  [unwired: 1 in, 1 out]
          }
        }
        n179 = call "AMC Destroy Message Queue.vi"("error in (no error)"=w358, "Message Queue in"=w360) -> ("error out"=w359:errorcluster)  [unwired: 9 out]
        n180 = call "IO.vi"("DO DATA"=bool[] [FALSE, FALSE, FALSE, FALSE, FALSE, FALSE, FALSE, FALSE] ("Writel_IO"), "IO Name"=string[] ["psu+   J3_1", "psu-   J3_5", "UART1_3V3  J63_1", "UART1_TX   J63_5", "UART1_RX   J63_6", "UART1_GND  J63_10", "PSU S+ J3_1", "PSU S- J3_5"], "IO?"=enum16{"DI", "DO"}."DO") -> ()  [unwired: 7 in, 2 out]
      }
    }
  }
